vi "Checksum.vi"(8 "Error In":errorcluster, 10 "Packet":u8[](array[numeric]), 11 "LINX Device Config":T1) -> (0 "Error Out":errorcluster, 1 "Checksum Pass?":bool, 2 "Packet":u8[](array[numeric]), 3 "LINX Device Config":T1)   [LabVIEW 2014, in "LMH-LINX.lvlib" / "Device.lvlib"]
uses:
  <vilib>/MakerHub/LINX/Private/Device/Device.lvlib
  <vilib>/MakerHub/LINX/Private/Device/Type Defs/LINX Device Config.ctl
  <vilib>/MakerHub/LINX/Private/Type Defs/Interface.ctl
  <vilib>/MakerHub/LINX/Private/Device/Type Defs/TCP Config.ctl
  <vilib>/MakerHub/LINX/Private/Device/Type Defs/Channels.ctl
  <vilib>/MakerHub/LINX/LMH-LINX.lvlib
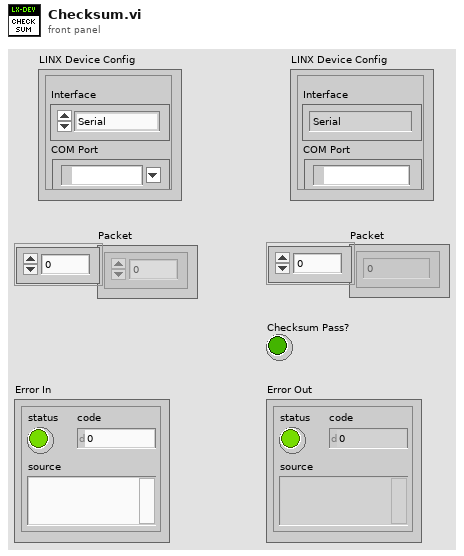
[diagram p1: front panel]
types:
  T1 = typedef "LMH-LINX.lvlib/Device.lvlib/LINX Device Config.ctl" = cluster{"Interface":T2, "COM Port":refnum<visa-resource-name>, "TCP Configuration":T3, "Device Family":u8, "Device ID":u8, "Device Name":string, "TCP Ref":refnum<k5>, "Channels":T4}
  T2 = typedef "LMH-LINX.lvlib/Interface.ctl" = enum16{"Serial", "TCP"}
  T3 = typedef "LMH-LINX.lvlib/Device.lvlib/TCP Config.ctl" = cluster{"IP Address":string, "Port":u16}
  T4 = typedef "LMH-LINX.lvlib/Channels.ctl" = cluster{"DI":u8[], "DO":u8[], "AI":u8[], "AO":u8[], "PWM":u8[], "QE":u8[], "UART":u8[], "I2C 2":u8[], "SPI":u8[], "CAN":u8[], "Servo":u8[], "AI Ref (V)":dbl, "AI Resolution (Bits)":u8, "AO Ref (V)":dbl, "AO Resolution (Bits)":u8}
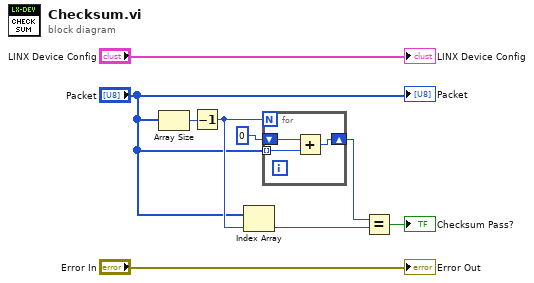
[diagram p0: block diagram]
diagram:
  n1 = Array Size(array="Packet") -> (size(s)=w9:i32)
  n2 = Decrement(x=w9) -> (x-1=w8:i32)
  n3 = Index Array(array="Packet", index=w8) -> (element=w7:u8)
  n4 = for {
    N: w8 -> [_]
    tunnel: "Packet" -> [w11] mode=indexing
    shift-right: [w10] -> w5
    shift-left: u8 0 -> [w12]
    n5 = Add(x=w12, y=w11) -> (x+y=w10:u8)
  }
  n6 = Equal?(x=w5, y=w7) -> (x = y?=→"Checksum Pass?":bool)
  "Packet" <- "Packet"
  "Error Out" <- "Error In"
  "LINX Device Config" <- "LINX Device Config"
